vi "Append Timeout.vi"(0 "State in":refnum<class "State.lvclass">, 7 "Timeout":refnum<class "Timeout.lvclass">, 11 "error in (no error)":errorcluster) -> (4 "State out":refnum<class "State.lvclass">, 15 "error out":errorcluster)   [LabVIEW 2015, in "State.lvclass"]
uses:
  State.lvclass
  Timeout/Timeout.lvclass
  State.lvclass/State.ctl
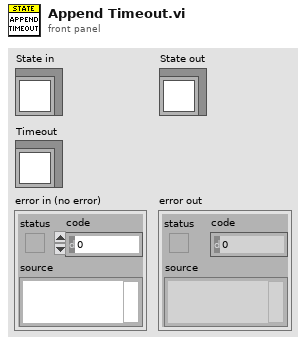
[diagram p1: front panel]
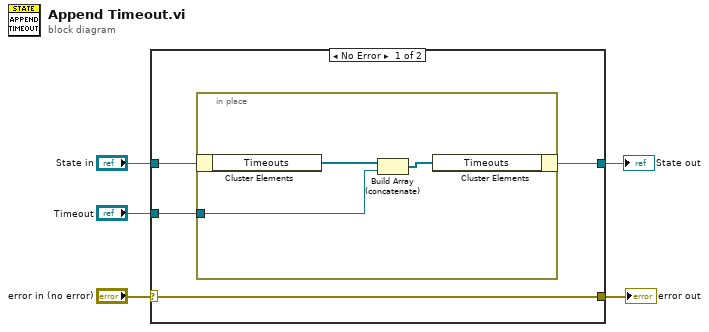
[diagram p0: block diagram]
diagram:
  n1 = case shown="No Error" "error in (no error)" {
    selector: "error in (no error)" -> [w9 w14]
    tunnel: [w9 w14] -> w4
    tunnel: "State in" -> [w8 w13]
    tunnel: [w7 w13] -> w2
    tunnel: "Timeout" -> [w6 _]
    frame No Error {
      n2 = in-place {
        in-place-border: w6 -> [w11]
        n3 = in-place-cluster #1(w8) -> ("Timeouts"=w12:refnum<class "Timeout.lvclass">[])
        n4 = Build Array (concatenate)(w12, w11) -> (w10:refnum<class "Timeout.lvclass">[])
        n5 = in-place-cluster #1("Timeouts"=w10) -> (w7:refnum<class "State.lvclass">)
      }
    }
    frame Error {
    }
  }
  "error out" <- w4
  "State out" <- w2
